vi "Test Proxy.vi"() -> ()   [LabVIEW 2020]
uses:
  <vilib>/httpClient/LabVIEWHTTPClient.lvlib
  <vilib>/JDP Science/JSONtext/JSONtext.lvlib
panel:
  out "body":string
  out "Status":string
  out "error out":errorcluster
  in  "error in":errorcluster
  in  "Node":string="4hzsj"
  in  "Token":string
  in  "OSF API URL":string="https://api.osf.io/v2/"
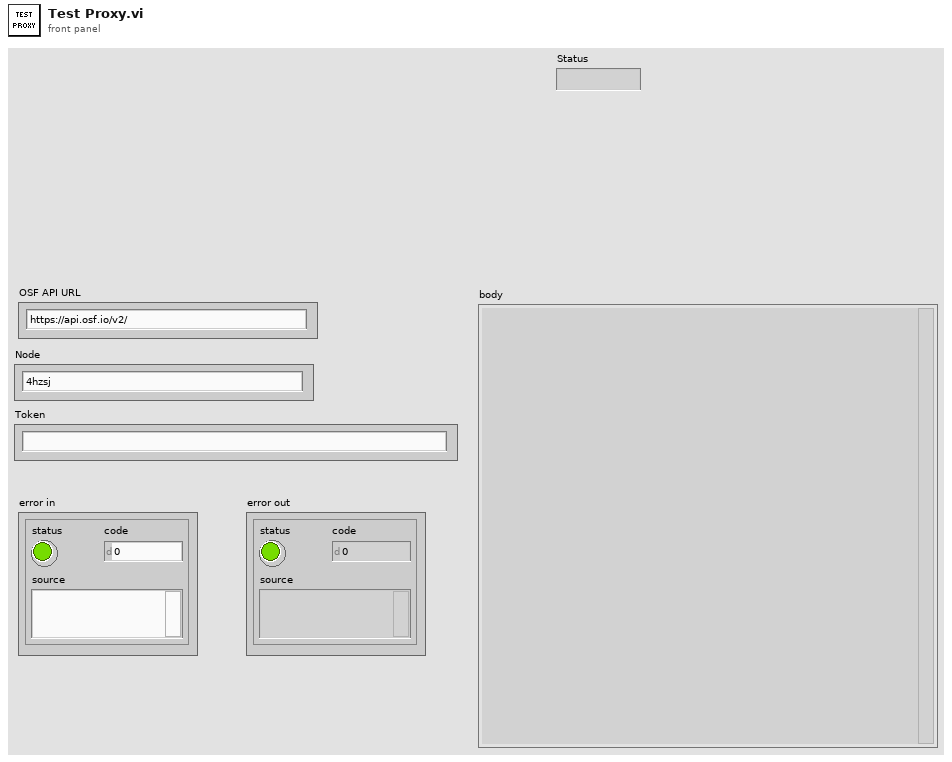
[diagram p1: front panel]
types:
  T1 = typedef "LabVIEWHTTPClient.lvlib/ClientHandle.ctl" = refnum<k1>
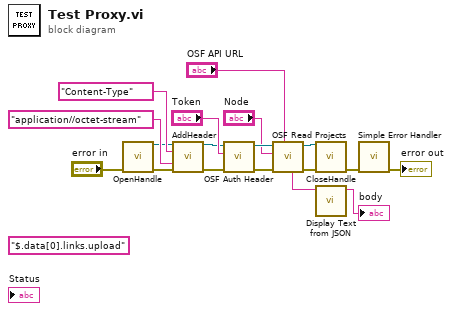
[diagram p0: block diagram]
diagram:
  (unwired) "$.data[0].links.upload" ("$Path or Item Name")
  n1 = call <vilib>:"OpenHandle.vi"("error in (no error)"="error in") -> ("client handle out"=w15:T1, "error out"=w16:errorcluster)  [unwired: 13 in]
  n2 = call <vilib>:"AddHeader.vi"("client handle"=w15, "header"="Content-Type", "value"="application//octet-stream", "error in (no error)"=w16) -> ("client handle out"=w11:T1, "error out"=w13:errorcluster)  [unwired: 10 in]
  n3 = call "OSF Auth Header.vi"("error in"=w13, "Token"="Token", "client handle"=w11) -> ("error out"=w10:errorcluster, "client handle out"=w9:T1)  [unwired: 7 in]
  n4 = call "OSF Read Projects.vi"("OSF API URL"="OSF API URL", "error in"=w10, "node"="Node", "client handle"=w9) -> ("error out"=w6:errorcluster, "client handle out"=w5:T1, "body"=w3:string)  [unwired: 2 in, 3 out]
  n5 = call <vilib>:"CloseHandle.vi"("client handle"=w5, "error in (no error)"=w6) -> ("error out"=w7:errorcluster)  [unwired: 13 in]
  n6 = call <vilib>:"Display Text from JSON.vi"("Input JSON"=w3) -> ("Display Text"=→"body":string)  [unwired: 8 in, 2 out]
  n7 = call <vilib>:"Simple Error Handler.vi"("error in (no error)"=w7) -> ("error out"=→"error out":errorcluster)  [unwired: 4 in, 4 out]
